vi "AnaliseStatusInversor.vi"(8 "error in":errorcluster) -> (0 "error out":errorcluster, 2 "InfoStatus":string, 3 "DadosInversor":T1(array[cluster]))   [LabVIEW 2019]
uses:
  VariaveisMedicao.vi
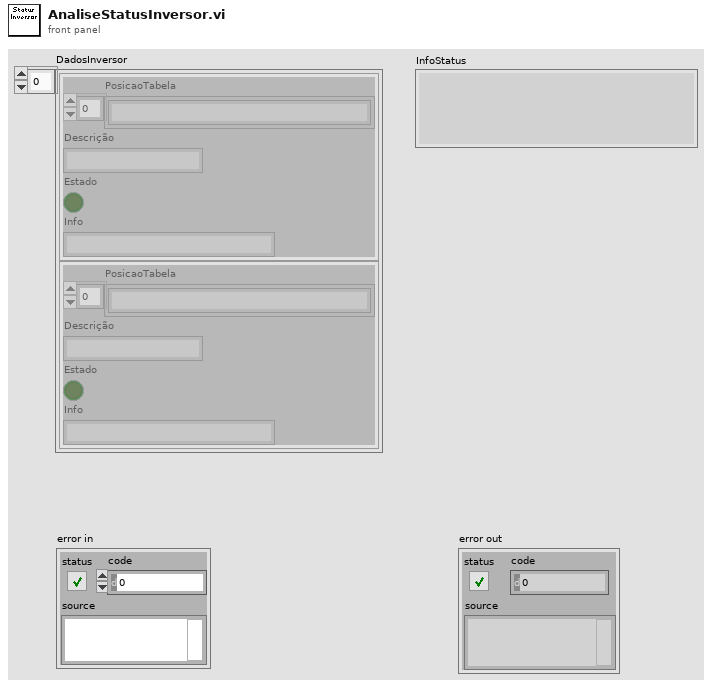
[diagram p1: front panel]
types:
  T1 = cluster{"PosicaoTabela":string[], "Descrição":string, "Estado":bool, "Info":string}[]
  T2 = cluster{"Memoria":string, "TabelaPosicoesMemoria":string[][], "Status":bool[]}[]
  T3 = cluster{"PosicaoTabela":string[], "Descrição":string, "Estado":bool, "Info":string}
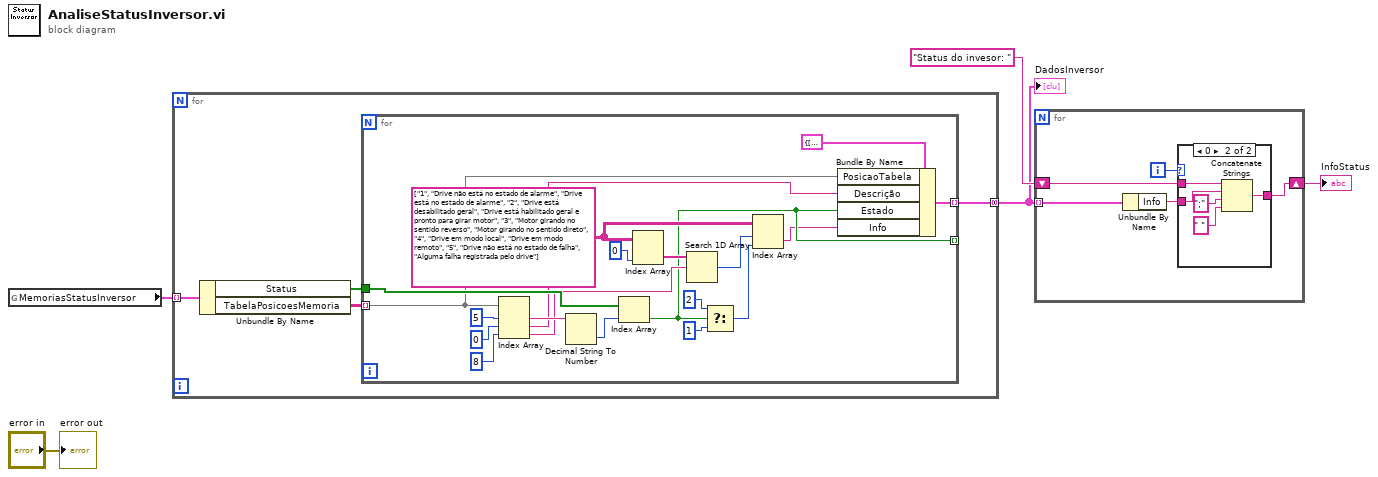
[diagram p0: block diagram]
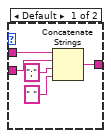
[diagram p2: hidden frame]
diagram:
  n1 = global read "VariaveisMedicao.vi" "MemoriasStatusInversor"() -> (w5:T2)
  n2 = for {
    tunnel: w5 -> [w9] mode=indexing
    tunnel: [w6] -> w2 mode=concatenating
    n3 = Unbundle By Name(w9) -> ("Status"=w7:bool[], "TabelaPosicoesMemoria"=w8:string[][])
    n4 = for {
      tunnel: w8 -> [w24] mode=indexing
      tunnel: w7 -> [w28]
      tunnel: [w14] -> _ mode=indexing
      tunnel: [w21] -> w6 mode=indexing
      w16 = string[][] [["1", "Drive não está no estado de alarme", "Drive está no estado de alarme"], ["2", "Drive está desabilitado geral", "Drive está habilitado geral e pronto para girar motor"], ["3", "Motor girando no sentido reverso", "Motor girando no sentido direto"], ["4", "Drive em modo local", "Drive em modo remoto"], ["5", "Drive não está no estado de falha", "Alguma falha registrada pelo drive"]]
      n5 = Index Array(array=w24, index #1=5 ("index"), index #2=0 ("index"), index #3=8 ("index")) -> (element #1=w27:string, element #2=w22:string, element #3=w17:string)
      n6 = Decimal String To Number(string=w27) -> (number=w26:i32)  [unwired: 2 in, 1 out]
      n7 = Index Array(array=w28, index=w26) -> (element=w14:bool)
      n8 = Index Array(array=w16, index (col)=0 ("disabled index (col)")) -> (element=w18:string[])  [unwired: 1 in]
      n9 = Search 1D Array(1D array=w18, element=w17) -> (index of element=w15:i32)  [unwired: 1 in]
      n10 = Select(t=2, s=w14, f=1) -> (s? t:f=w11:i32)
      n11 = Index Array(array=w16, index (row)=w15, index (col)=w11) -> (element=w10:string)
      n12 = Bundle By Name(cluster=T3 {"PosicaoTabela"=[], "Descrição"="", "Estado"=FALSE, "Info"=""} ("Cluster"), "PosicaoTabela"=w24, "Descrição"=w22, "Estado"=w14, "Info"=w10) -> (w21:T3)
    }
  }
  "DadosInversor" <- w2
  n13 = for {
    shift-right: [w31] -> w1
    shift-left: "Status do invesor: " -> [w30]
    tunnel: w2 -> [w34] mode=indexing
    i -> [w33]
    n14 = Unbundle By Name(w34) -> ("Info"=w32:string)
    n15 = case shown="0" w33 {
      tunnel: w32 -> [w38 w44]
      tunnel: [w35 w41] -> w31
      tunnel: w30 -> [w39 w40]
      frame Default {
        n16 = Concatenate Strings(w39, w38, ";" ("string"), " " ("string")) -> (w35:string)
      }
      frame 0 {
        n17 = Concatenate Strings(w40, w44, ";" ("string"), " " ("string")) -> (w41:string)
      }
    }
  }
  "InfoStatus" <- w1
  "error out" <- "error in"
